vi "Compare Images Radial.vi"(10 "Image 2":path=path "C:/Users/Matthew/Clients/Users Group/Coding Challenge/Submissions/drt_altered.bmp", 11 "Image 1":path=path "C:/Users/Matthew/Clients/Users Group/Coding Challenge/Submissions/drt.bmp") -> (3 "Perceptual Cross Correlation":dbl)   [LabVIEW 2015, in "Perceptual Hash Comparison.lvclass"]
doc: "This VI calls the pHash DLL. It requires that the images are BMPs."
uses:
  Perceptual Hash Comparison.lvclass
  Image Comparison/Image Comparison.lvclass
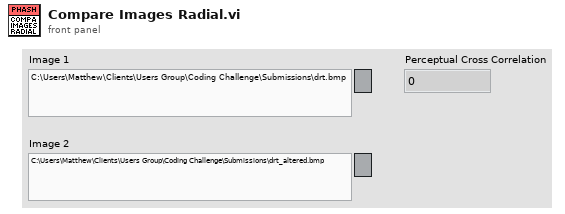
[diagram p1: front panel]
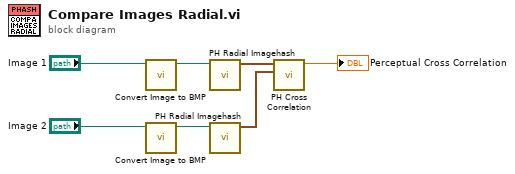
[diagram p0: block diagram]
diagram:
  n1 = call "Convert Image to BMP.vi"("Image Path in"="Image 1") -> ("BMP Image Path out"=w3:path)  [unwired: 9 in, 1 out]
  n2 = call "Convert Image to BMP.vi"("Image Path in"="Image 2") -> ("BMP Image Path out"=w1:path)  [unwired: 9 in, 1 out]
  n3 = call "PH Radial Imagehash.vi"("Image Path"=w3) -> ("Digest"=w7:cluster{"*id":u32, "*Coeffs":u32, "size":i32})  [unwired: 10 in]
  n4 = call "PH Radial Imagehash.vi"("Image Path"=w1) -> ("Digest"=w6:cluster{"*id":u32, "*Coeffs":u32, "size":i32})  [unwired: 10 in]
  n5 = call "PH Cross Correlation.vi"("Digest 2"=w6, "Digest 1"=w7) -> ("Perceptual Cross Correlation"=→"Perceptual Cross Correlation":dbl)  [unwired: 9 in]
